vi "Write field values.vi"(8 "error in (no error)":errorcluster, 10 "field values":variant, 11 "DbMeasurement in":refnum<class "DbMeasurement.lvclass">) -> (0 "error out":errorcluster, 3 "DbMeasurement out":refnum<class "DbMeasurement.lvclass">)   [LabVIEW 2013, in "DbMeasurement.lvclass"]
doc: "This accessor enqueues field values into the field values queue."
uses:
  DbMeasurement.lvclass
  DbMeasurement.lvclass/DbMeasurement.ctl
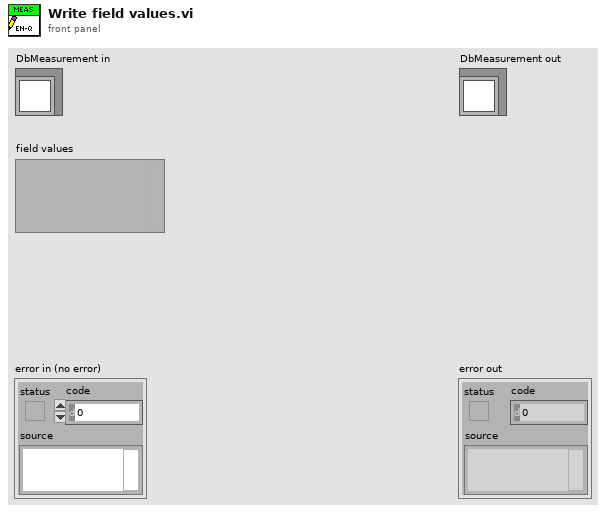
[diagram p1: front panel]
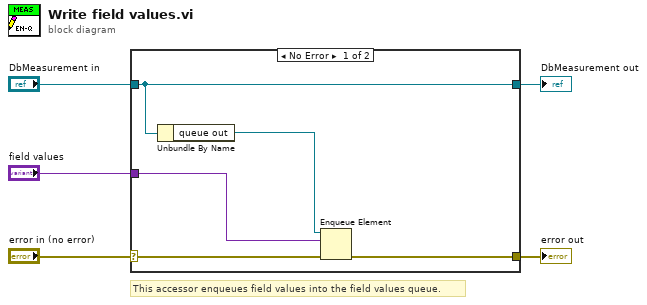
[diagram p0: block diagram]
diagram:
  # "This accessor enqueues field values into the field values queue."
  n1 = case shown="No Error" "error in (no error)" {
    selector: "error in (no error)" -> [w10 w11]
    tunnel: [w9 w11] -> w4
    tunnel: [w6 w12] -> w2
    tunnel: "DbMeasurement in" -> [w6 w12]
    tunnel: "field values" -> [w7 _]
    frame No Error {
      n2 = Unbundle By Name(w6) -> ("queue out"=w8:refnum<queue>)
      n3 = Enqueue Element(queue=w8, element=w7, error in (no error)=w10) -> (error out=w9:errorcluster)  [unwired: 1 in, 2 out]
    }
    frame Error {
    }
  }
  "error out" <- w4
  "DbMeasurement out" <- w2
